vi "Find all dependencies of all vis in memory.vi"(4 "error in":errorcluster, 7 "All VIs in .proj":string[](array[string])) -> (0 "error out":errorcluster, 2 "Dependencies":string[](array[string]))   [LabVIEW 2010]
doc: "This .vi finds a list of all of the dependencies of the .vis in memory that are not present in the project vis."
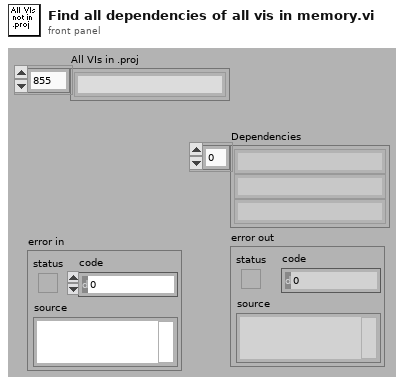
[diagram p1: front panel]
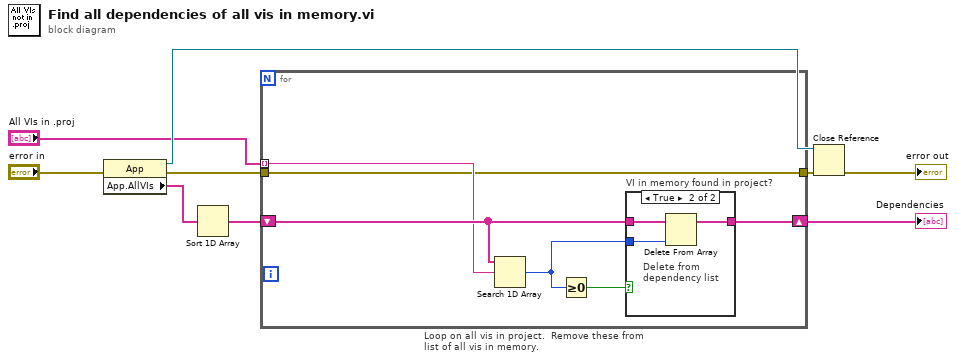
[diagram p0: block diagram]
diagram:
  n1 = property class="App"(error in="error in") -> (reference out=w2:refnum<vi>, error out=w5:errorcluster, "App.AllVIs"=w9:string[])  [unwired: 1 in]
  n2 = Sort 1D Array(array=w9) -> (sorted array=w7:string[])
  n3 = for "Loop on all vis in project.  Remove these from list of all vis in memory." {
    tunnel: "All VIs in .proj" -> [w11] mode=indexing
    shift-right: [w12] -> w8
    shift-left: w7 -> [w13]
    tunnel: w5 -> [w10]
    tunnel: [w10] -> w4
    n4 = Search 1D Array(1D array=w13, element=w11) -> (index of element=w14:i32)  [unwired: 1 out]
    n5 = Greater Or Equal To 0?(x=w14) -> (x >= 0?=w15:bool)
    n6 = case "VI in memory found in project?" shown="True" w15 {
      tunnel: w14 -> [_ w19]
      tunnel: w13 -> [w16 w18]
      tunnel: [w16 w17] -> w12
      frame False {
      }
      frame True {
        # "Delete from \ndependency list"
        n7 = Delete From Array(array=w18, index=w19) -> (array with subset deleted=w17:string[])  [unwired: 1 in, 1 out]
      }
    }
  }
  "Dependencies" <- w8
  n8 = Close Reference(reference=w2, error in (no error)=w4) -> (error out=→"error out":errorcluster)
